vi "MCAWindow.vi"(10 "Histogram Data":u32[][](array[numeric]), 11 "Window":i32[](array[numeric])) -> (1 "Ch1 Counts":u32=199, 3 "Ch0 Counts":u32=198)   [LabVIEW 2013]
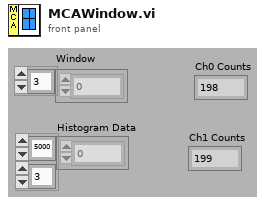
[diagram p1: front panel]
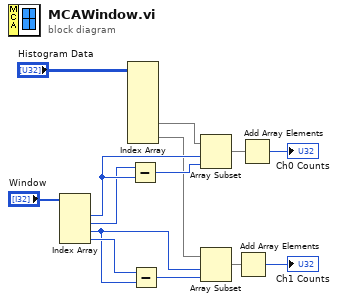
[diagram p0: block diagram]
diagram:
  n1 = Index Array(array="Window") -> (element #1=w6:i32, element #2=w5:i32, element #3=w1:i32, element #4=w2:i32)  [unwired: 4 in]
  n2 = Index Array(array="Histogram Data") -> (element #3=w3:u32[], element #4=w4:u32[])  [unwired: 8 in, 2 out]
  n3 = Subtract(x=w5, y=w6) -> (x-y=w9:i32)
  n4 = Subtract(x=w2, y=w1) -> (x-y=w12:i32)
  n5 = Array Subset(array=w3, index=w6, length=w9) -> (w10:u32[])
  n6 = Array Subset(array=w4, index=w1, length=w12) -> (w13:u32[])
  n7 = Add Array Elements(numeric array=w13) -> (sum=→"Ch1 Counts":u32)
  n8 = Add Array Elements(numeric array=w10) -> (sum=→"Ch0 Counts":u32)
